vi "test-MecaDrvPoseEst2-Test2.vi"(8 "error in (no error)":errorcluster) -> (0 "error out":errorcluster, 3 "Test Passed":bool)   [LabVIEW 2019]
uses:
  <vilib>/Rock Robotics/WPI/ThirdParty/JAS_Junk/TrajLib/Rotation2d_CreateAngle.vi
  <vilib>/Rock Robotics/WPI/ThirdParty/JAS_Junk/TrajLib/MatBuilder_Create.vi
  <vilib>/Rock Robotics/WPI/ThirdParty/JAS_Junk/TrajLib/Pose2d_TransformBy.vi
  <vilib>/Rock Robotics/WPI/ThirdParty/JAS_Junk/TrajLib/Translation2d_RotateBy.vi
  <vilib>/Rock Robotics/WPI/ThirdParty/JAS_Junk/TrajLib/Translation2d_Plus.vi
  <vilib>/Rock Robotics/WPI/ThirdParty/JAS_Junk/TrajLib/Rotation2d_Plus.vi
  <vilib>/Rock Robotics/WPI/ThirdParty/JAS_Junk/TrajLib/Pose2d_New_TRRO.vi
  <vilib>/Rock Robotics/WPI/ThirdParty/JAS_Junk/TrajLib/Rotation2d_RotateBy.vi
  <vilib>/Rock Robotics/WPI/ThirdParty/JAS_Junk/TrajLib/Rotation2d_CreateXY.vi
  <vilib>/Rock Robotics/WPI/ThirdParty/JAS_Junk/TrajLib/Util_CalcDist.vi
  <vilib>/Rock Robotics/WPI/ThirdParty/JAS_Junk/TrajLib/Trajectory_Library.lvlib
panel:
  out "max x error":dbl
  out "max y err":dbl
  out "Y Error":dbl[](array[numeric])
  out "X error":dbl[](array[numeric])
  out "Total":i32
  out "Total passed":i32
  out "Sub error":bool
  out "End Y pos passed":bool
  out "End X pos passed":bool
  out "AddVisionCount":i32
  out "TotalTImeSecs 2":dbl
  out "BenchProcessing \nTimer Per Pass":dbl
  out "BenchTotalTime":dbl
  out "BenchTotalPasses":dbl
  out "MaxErrPassed":bool
  out "MeanPassed":bool
  out "ErrorSumNormalized":dbl
  out "Error Sum":dbl
  out "Max Error":dbl
  out "VIsionMeasCount":i32
  out "TotalTImeSecs":dbl
  out "Position Graph":cluster{dbl[], dbl[]}[](graph)
  out "PoseEst2NewErr":errorcluster
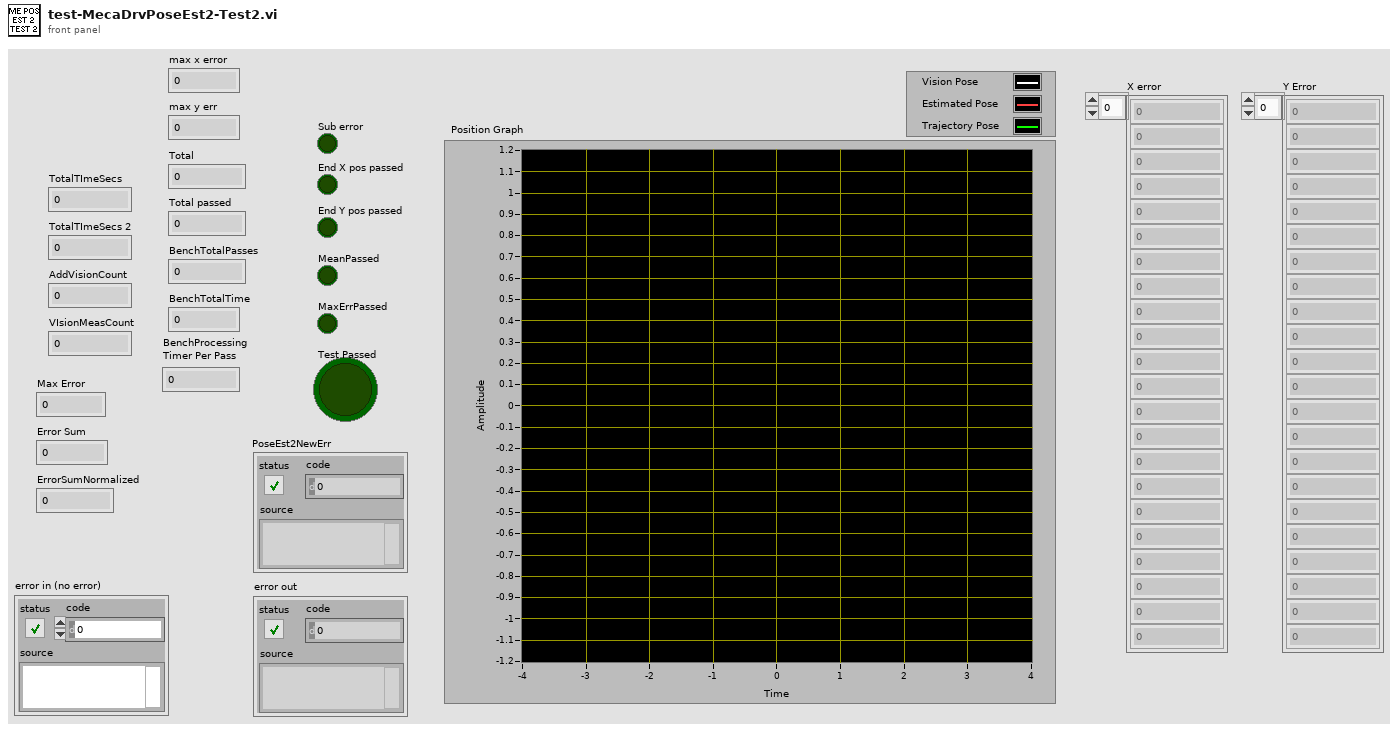
[diagram p1: front panel]
types:
  T1 = typedef "Trajectory_Library.lvlib/TRANSLATION2D.ctl" = cluster{"X":dbl, "Y":dbl}
  T2 = typedef "Trajectory_Library.lvlib/MECA_DRIVE_KINEMATICS.ctl" = cluster{"FrontLeft":T1, "FrontRight":T1, "RearLeft":T1, "RearRight":T1, "InverseKinematics":T3, "ForwardKinematics":T3, "PrevCoR":T1}
  T3 = typedef "NI_Matrix.lvlib/RealMatrix.ctl" = dbl[][]
  T4 = typedef "Trajectory_Library.lvlib/MECA_WHEEL_POSITIONS.ctl" = cluster{"FrontLeft":dbl, "FrontRight":dbl, "RearLeft":dbl, "RearRight":dbl, "P":bool}
  T5 = typedef "Trajectory_Library.lvlib/POSE2D.ctl" = cluster{"TRANSLATION":T1, "ROTATION":T6}
  T6 = typedef "Trajectory_Library.lvlib/ROTATION2D.ctl" = cluster{"VALUE":dbl, "COS":dbl, "SIN":dbl}
  T7 = typedef "Trajectory_Library.lvlib/TRAJ_CONFIG.ctl" = cluster{"MaxVelocity":dbl, "Max Acceleration":dbl, "StartVelocity":dbl, "End Velocity":dbl, "Reversed":bool, "Constraints":variant[]}
  T8 = typedef "Trajectory_Library.lvlib/MECA_DRIVE_POSE_EST2.ctl" = cluster{"M_Vision_K":T3, "m_nominal_dT":dbl, "m_PrevTime_Sec":dbl, "Pose_Buffer":T9, "Meca_Drive_Odom":T10, "M_Q":T3}
  T9 = typedef "Trajectory_Library.lvlib/TIME_INTERPOLATABLE_VARIANT.ctl" = cluster{"TimeStamps":dbl[], "DataArray":variant[], "Min_TimeStamp":dbl, "Max_TimeStamp":dbl, "ItemCount":i32, "MaxBufferTime":dbl}
  T10 = typedef "Trajectory_Library.lvlib/MECA_DRIVE_ODOMETRY.ctl" = cluster{"POSE":T5, "GyroOffset":T6, "PreviousAngle":T6, "Kinematics":T2, "PreviousWheelPositions":T4}
  T11 = typedef "Trajectory_Library.lvlib/TRAJECTORY.ctl" = cluster{"TotalTImeSecs":dbl, "States":T12[]}
  T12 = typedef "Trajectory_Library.lvlib/TRAJ_STATE.ctl" = cluster{"TimeSeconds":dbl, "Velocity":dbl, "Acceleration":dbl, "POSE":T5, "Curvature":dbl}
  T13 = typedef "Trajectory_Library.lvlib/TRANSFORM2D.ctl" = cluster{"TRANSLATION":T1, "ROTATION":T6, "xF":bool}
  T14 = cluster{"MaxErrPassed":bool, "MeanPassed":bool, "Error Sum":dbl, "ErrorSumNormalized":dbl, "Max Error":dbl, "AddVisionCount":i32, "VIsionApplyCount":i32, "BenchTotalPasses":dbl, "BenchTotalTime":dbl, "BenchProcessing \nTimer Per Pass":dbl, "TotalTImeSecs":dbl, "End X pos passed":bool, "End Y pos passed":bool, "Sub error":bool, "End X Dev":dbl, "End Y Dev":dbl}
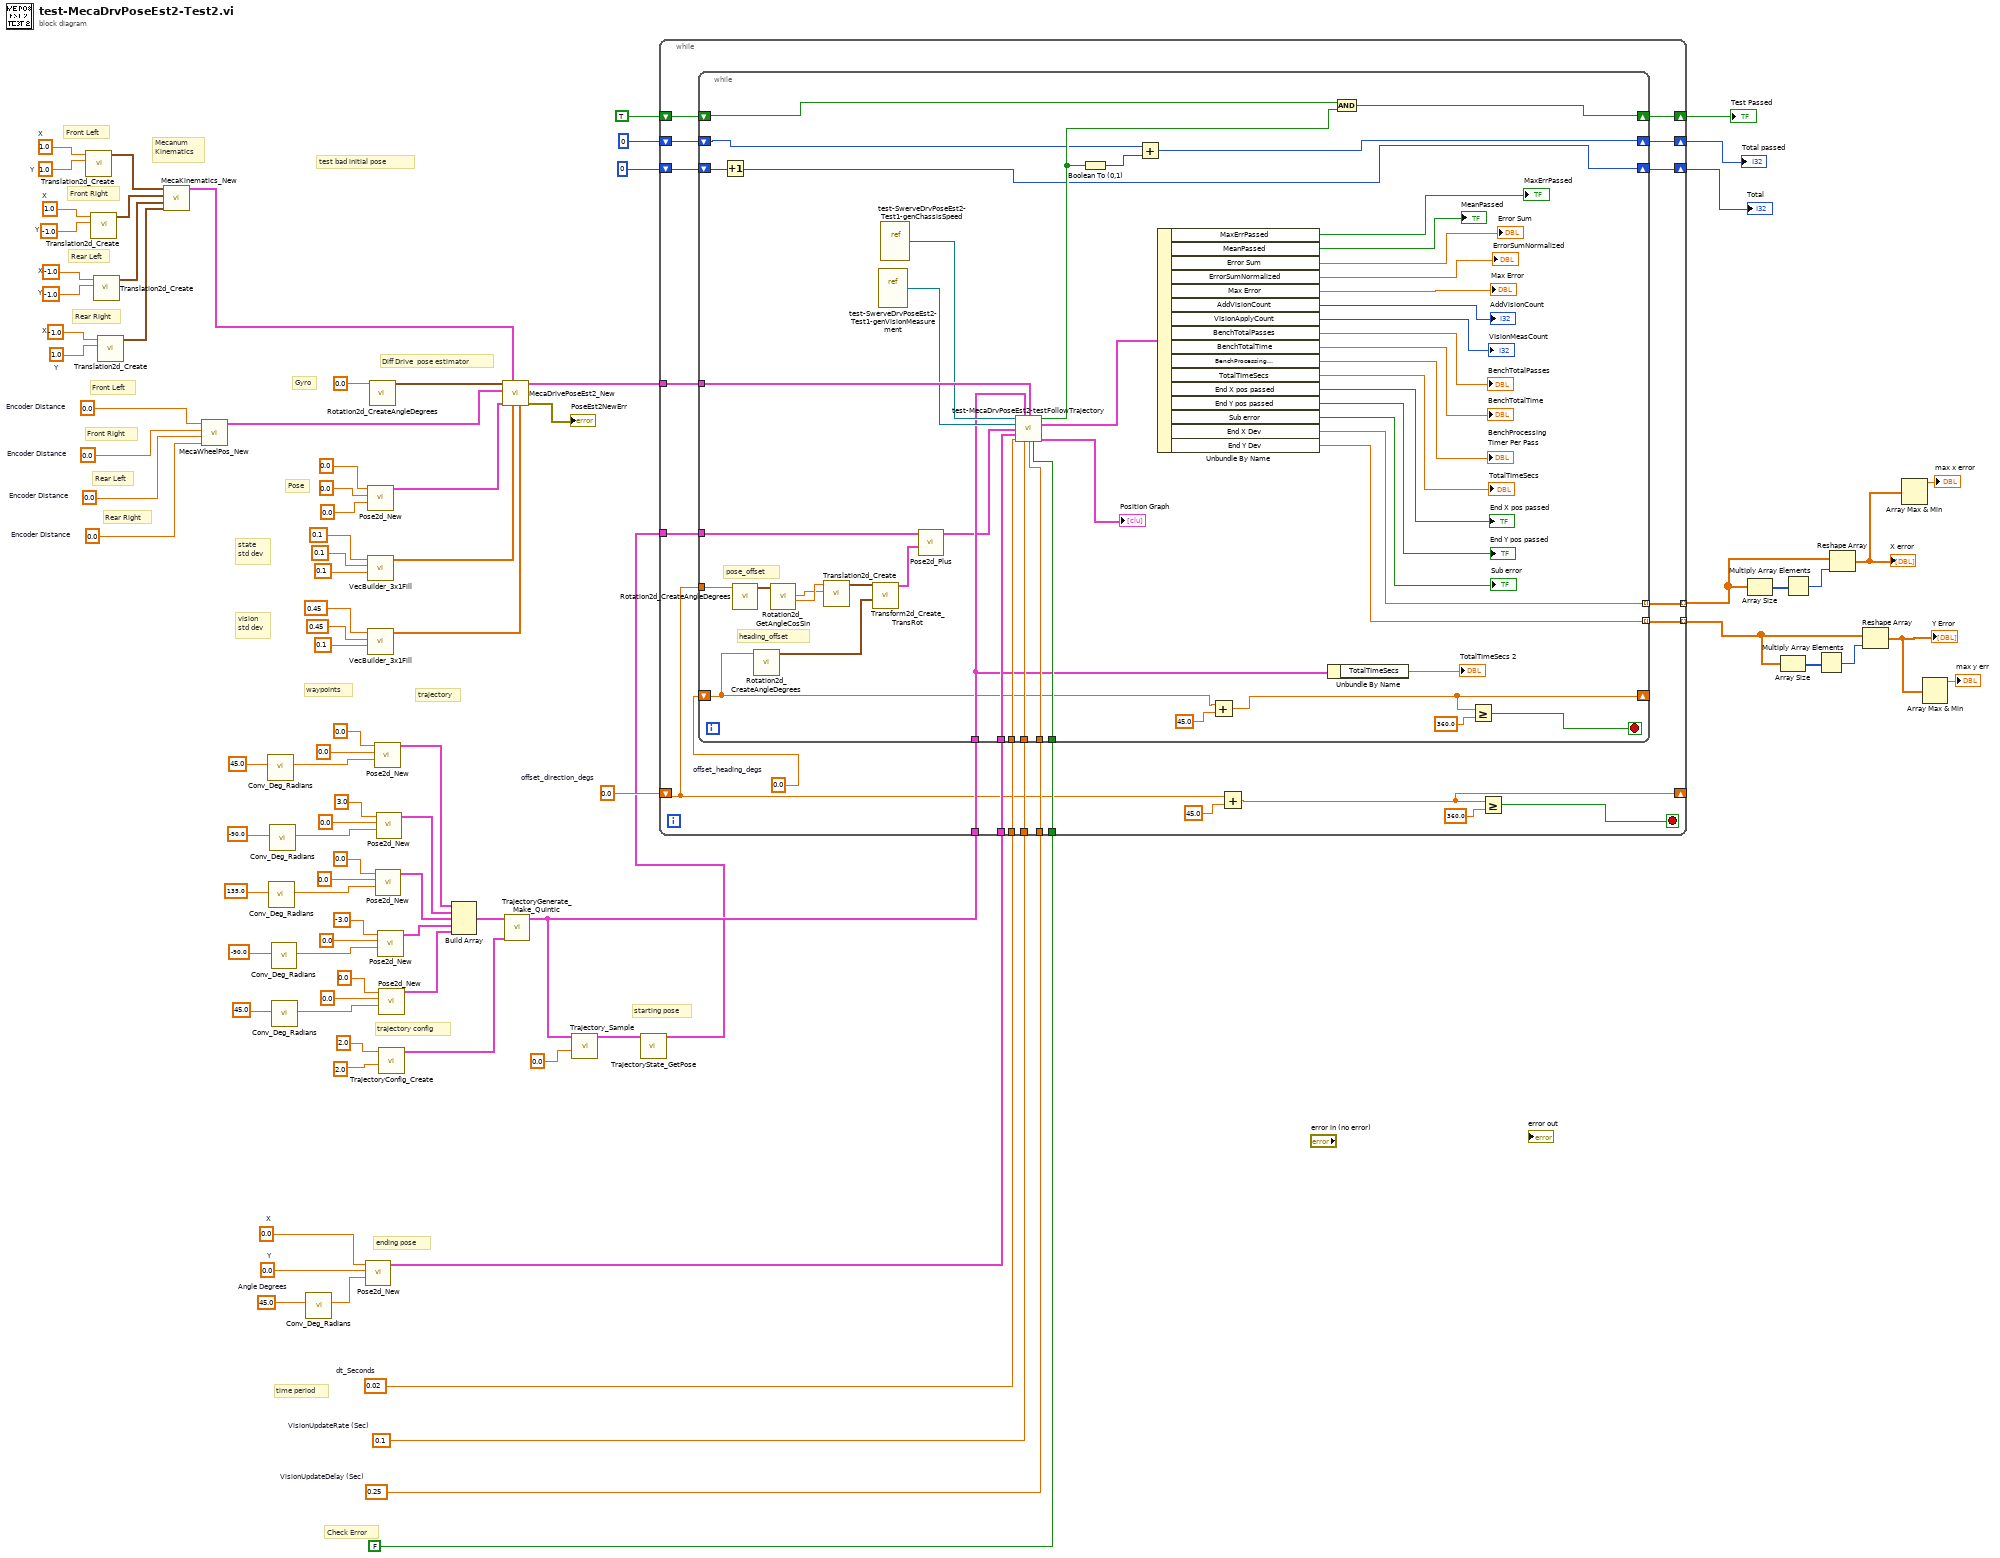
[diagram p0: block diagram]
diagram:
  w10 = -1.0  # X
  w9 = 1.0  # Y
  w8 = -1.0  # X
  w7 = -1.0  # Y
  w6 = 1.0  # X
  w5 = -1.0  # Y
  w4 = 1.0  # X
  w3 = 1.0  # Y
  w15 = 0.0  # Encoder Distance
  w16 = 0.0  # Encoder Distance
  w17 = 0.0  # Encoder Distance
  w18 = 0.0  # Encoder Distance
  w36 = 0.0  # offset_direction_degs
  w41 = 0.25  # VisionUpdateDelay (Sec)
  w42 = 0.1  # VisionUpdateRate (Sec)
  w47 = 0.0  # X
  w46 = 0.0  # Y
  w44 = 45.0  # Angle Degrees
  w48 = 0.02  # dt_Seconds
  # "Mecanum\nKinematics"
  # "Rear Right"
  # "Rear Left"
  # "Front Right"
  # "Front Left"
  # "Front Left"
  # "Rear Right"
  # "Rear Left"
  # "Front Right"
  # "test bad initial pose"
  # "starting pose"
  # "Check Error"
  # "ending pose"
  # "state \nstd dev"
  # "time period"
  # "vision \nstd dev"
  # "Pose"
  # "Gyro"
  # "Diff Drive  pose estimator"
  # "trajectory config"
  # "trajectory"
  # "waypoints"
  n1 = call <vilib>:"Translation2d_Create.vi"("Y"=w3, "X"=w4) -> ("TRANSLATION"=w11:T1)  [unwired: 9 in]
  n2 = call <vilib>:"Translation2d_Create.vi"("Y"=w5, "X"=w6) -> ("TRANSLATION"=w12:T1)  [unwired: 9 in]
  n3 = call <vilib>:"Translation2d_Create.vi"("Y"=w7, "X"=w8) -> ("TRANSLATION"=w13:T1)  [unwired: 9 in]
  n4 = call <vilib>:"Translation2d_Create.vi"("Y"=w9, "X"=w10) -> ("TRANSLATION"=w14:T1)  [unwired: 9 in]
  n5 = call <vilib>:"MecaKinematics_New.vi"("RearRight"=w14, "RearLeft"=w13, "FrontRight"=w12, "FrontLeft"=w11) -> ("MECA_DRIVE_KINEMATICS"=w1:T2)  [unwired: 7 in]
  n6 = call <vilib>:"MecaWheelPos_New.vi"("RearRightPosition"=w15, "RearLeftPosition"=w16, "FrontRightPosition"=w17, "FrontLeftPosition"=w18) -> ("MECA_WHEEL_POSITIONS"=w2:T4)  [unwired: 7 in]
  n7 = call <vilib>:"Conv_Deg_Radians.vi"("Degress"=45.0 ("Heading")) -> ("Radians"=w70:dbl)  [unwired: 10 in]
  n8 = call <vilib>:"Conv_Deg_Radians.vi"("Degress"=135.0 ("Heading")) -> ("Radians"=w78:dbl)  [unwired: 10 in]
  n9 = call <vilib>:"Conv_Deg_Radians.vi"("Degress"=-90.0 ("Heading")) -> ("Radians"=w74:dbl)  [unwired: 10 in]
  n10 = call <vilib>:"Conv_Deg_Radians.vi"("Degress"=-90.0 ("Heading")) -> ("Radians"=w82:dbl)  [unwired: 10 in]
  n11 = call <vilib>:"Conv_Deg_Radians.vi"("Degress"=45.0 ("Heading")) -> ("Radians"=w86:dbl)  [unwired: 10 in]
  n12 = call <vilib>:"Conv_Deg_Radians.vi"("Degress"=w44) -> ("Radians"=w45:dbl)  [unwired: 10 in]
  n13 = call <vilib>:"Pose2d_New.vi"("Heading"=w45, "Y"=w46, "X"=w47) -> ("out POSe"=w43:T5)  [unwired: 8 in]
  n14 = call <vilib>:"Pose2d_New.vi"("Heading"=0.0, "Y"=0.0, "X"=0.0) -> ("out POSe"=w56:T5)  [unwired: 8 in]
  n15 = call <vilib>:"VecBuilder_3x1Fill.vi"("R2"=0.1 ("element"), "R1"=0.1 ("element"), "R0"=0.1 ("element")) -> ("output matrix"=w51:T3)  [unwired: 8 in]
  n16 = call <vilib>:"VecBuilder_3x1Fill.vi"("R2"=0.1 ("element"), "R1"=0.45 ("element"), "R0"=0.45 ("element")) -> ("output matrix"=w50:T3)  [unwired: 8 in]
  n17 = call <vilib>:"Rotation2d_CreateAngleDegrees.vi"("Angle_Degrees"=0.0) -> ("ROTATION"=w55:T6)  [unwired: 10 in]
  n18 = call <vilib>:"Pose2d_New.vi"("Heading"=w70, "Y"=0.0, "X"=0.0) -> ("out POSe"=w69:T5)  [unwired: 8 in]
  n19 = call <vilib>:"Pose2d_New.vi"("Heading"=w78, "Y"=0.0, "X"=0.0) -> ("out POSe"=w66:T5)  [unwired: 8 in]
  n20 = call <vilib>:"Pose2d_New.vi"("Heading"=w74, "Y"=0.0, "X"=3.0) -> ("out POSe"=w67:T5)  [unwired: 8 in]
  n21 = call <vilib>:"Pose2d_New.vi"("Heading"=w82, "Y"=0.0, "X"=-3.0) -> ("out POSe"=w65:T5)  [unwired: 8 in]
  n22 = call <vilib>:"Pose2d_New.vi"("Heading"=w86, "Y"=0.0, "X"=0.0) -> ("out POSe"=w91:T5)  [unwired: 8 in]
  n23 = call <vilib>:"TrajectoryConfig_Create.vi"("MaxAcceleration"=2.0, "MaxVelocity"=2.0) -> ("TRAJECTORY_CONFIG"=w88:T7)  [unwired: 9 in]
  n24 = Build Array(w69, w67, w66, w65, w91) -> (w89:T5[])
  n25 = call <vilib>:"MecaDrivePoseEst2_New.vi"("VisionMeasurementStdDevs"=w50, "StateStdDevs"=w51, "MECA_DRIVE_KINEMATICS"=w1, "InitialPose"=w56, "Module Positions"=w2, "gyroAngle"=w55) -> ("Error"=→"PoseEst2NewErr":errorcluster, "MecaDrivePoseEstimate"=w49:T8)  [unwired: 4 in]
  n26 = call <vilib>:"TrajectoryGenerate_Make_Quintic.vi"("traj_config"=w88, "waypointPOSE"=w89) -> ("TRAJECTORY"=w39:T11)  [unwired: 8 in, 1 out]
  n27 = call <vilib>:"Trajectory_Sample.vi"("Time"=0.0, "InputTRAJECTORY"=w39) -> ("OutputTRAJ_STATE"=w37:T12)  [unwired: 9 in]
  n28 = call <vilib>:"TrajectoryState_GetPose.vi"("TRAJ_STATE"=w37) -> ("TrajStatePose"=w35:T5)  [unwired: 10 in]
  n29 = while {
    tunnel: w49 -> [w115]
    tunnel: w48 -> [w114]
    tunnel: w43 -> [w113]
    tunnel: w42 -> [w112]
    tunnel: w41 -> [w111]
    tunnel: FALSE -> [w110]
    tunnel: w39 -> [w109]
    shift-right: [w104] -> _
    shift-left: w36 -> [w102]
    tunnel: w35 -> [w103]
    shift-right: [w100] -> w33
    shift-left: TRUE -> [w101]
    shift-right: [w98] -> w31
    shift-left: 0 -> [w99]
    shift-right: [w96] -> w29
    shift-left: 0 -> [w97]
    tunnel: [w95] -> w27 mode=indexing
    tunnel: [w94] -> w23 mode=indexing
    stop <- w106 stop-if-true
    w105 = 0.0  # offset_heading_degs
    n30 = while {
      tunnel: w115 -> [w165]
      tunnel: w114 -> [w164]
      tunnel: w113 -> [w163]
      tunnel: w112 -> [w162]
      tunnel: w111 -> [w161]
      tunnel: w110 -> [w159]
      tunnel: w109 -> [w141]
      shift-right: [w136] -> _
      shift-left: w105 -> [w134]
      tunnel: w103 -> [w127]
      tunnel: w102 -> [w132]
      shift-right: [w124] -> w100
      shift-left: w101 -> [w125]
      shift-right: [w120] -> w98
      shift-left: w99 -> [w122]
      shift-right: [w118] -> w96
      shift-left: w97 -> [w119]
      tunnel: [w117] -> w95 mode=indexing
      tunnel: [w116] -> w94 mode=indexing
      stop <- w137 stop-if-true
      # "heading_offset"
      # "pose_offset"
      n31 = Increment(x=w119) -> (x+1=w118:i32)
      n32 = call <vilib>:"Rotation2d_CreateAngleDegrees.vi"("Angle_Degrees"=w132) -> ("ROTATION"=w133:T6)  [unwired: 10 in]
      n33 = call <vilib>:"Rotation2d_CreateAngleDegrees.vi"("Angle_Degrees"=w134) -> ("ROTATION"=w129:T6)  [unwired: 10 in]
      n34 = call <vilib>:"Rotation2d_GetAngleCosSin.vi"("in ROTATION"=w133) -> ("Cosine"=w131:dbl, "Sine"=w130:dbl)  [unwired: 8 in, 1 out]
      n35 = call <vilib>:"Translation2d_Create.vi"("Y"=w130, "X"=w131) -> ("TRANSLATION"=w135:T1)  [unwired: 9 in]
      n36 = call <vilib>:"Transform2d_Create_TransRot.vi"("ROTATION"=w129, "TRANSLATION"=w135) -> ("TRANSFORM"=w128:T13)  [unwired: 9 in]
      n37 = vi-ref "test-SwerveDrvPoseEst2-Test1-genVisionMeasurement.vi"() -> (w157:refnum<vi>)
      n38 = vi-ref "test-SwerveDrvPoseEst2-Test1-genChassisSpeed.vi"() -> (w158:refnum<vi>)
      n39 = call <vilib>:"Pose2d_Plus.vi"("other TRANSFORM"=w128, "in POSE"=w127) -> ("out POSE"=w126:T5)  [unwired: 9 in]
      n40 = call "test-MecaDrvPoseEst2-testFollowTrajectory.vi"("chassisSpeedsGenerator"=w158, "TRAJECTORY"=w141, "MecaDrivePoseEstimate2"=w165, "genVisionMeasurement"=w157, "StartingPose"=w126, "EndingPose"=w163, "dt_Seconds"=w164, "VisionUpdateRate"=w162, "VisionUpdateDelay"=w161, "CheckError"=w159) -> ("Test Passed"=w123:bool, "Output Data"=w155:T14, "DataForGraph"=→"Position Graph":cluster{dbl[], dbl[]}[])  [unwired: 3 in]
      n41 = Boolean To (0,1)(Boolean=w123) -> (0, 1=w121:i16)
      n42 = Add(x=w122, y=w121) -> (x+y=w120:i32)
      n43 = Unbundle By Name(w155) -> ("MaxErrPassed"=→"MaxErrPassed":bool, "MeanPassed"=→"MeanPassed":bool, "Error Sum"=→"Error Sum":dbl, "ErrorSumNormalized"=→"ErrorSumNormalized":dbl, "Max Error"=→"Max Error":dbl, "AddVisionCount"=→"AddVisionCount":i32, "VIsionApplyCount"=→"VIsionMeasCount":i32, "BenchTotalPasses"=→"BenchTotalPasses":dbl, "BenchTotalTime"=→"BenchTotalTime":dbl, "BenchProcessing \nTimer Per Pass"=→"BenchProcessing \nTimer Per Pass":dbl, "TotalTImeSecs"=→"TotalTImeSecs":dbl, "End X pos passed"=→"End X pos passed":bool, "End Y pos passed"=→"End Y pos passed":bool, "Sub error"=→"Sub error":bool, "End X Dev"=w117:dbl, "End Y Dev"=w116:dbl)
      n44 = Add(x=w134, y=45.0) -> (x+y=w136:dbl)
      n45 = Unbundle By Name(w141) -> ("TotalTImeSecs"=→"TotalTImeSecs 2":dbl)
      n46 = And(x=w125, y=w123) -> (x .and. y?=w124:bool)
      n47 = Greater Or Equal?(x=w136, y=360.0) -> (x >= y?=w137:bool)
    }
    n48 = Add(x=w102, y=45.0) -> (x+y=w104:dbl)
    n49 = Greater Or Equal?(x=w104, y=360.0) -> (x >= y?=w106:bool)
  }
  "Test Passed" <- w33
  "Total passed" <- w31
  "Total" <- w29
  n50 = Array Size(array=w27) -> (size(s)=w28:i32[])
  n51 = Array Size(array=w23) -> (size(s)=w25:i32[])
  n52 = Multiply Array Elements(1:w28) -> (0:w26:i32)
  n53 = Multiply Array Elements(1:w25) -> (0:w24:i32)
  n54 = Reshape Array(w27, w26) -> (w22:dbl[])
  "X error" <- w22
  n55 = Reshape Array(w23, w24) -> (w21:dbl[])
  "Y Error" <- w21
  n56 = Array Max & Min(array=w22) -> (max value=→"max x error":dbl)  [unwired: 3 out]
  n57 = Array Max & Min(array=w21) -> (max value=→"max y err":dbl)  [unwired: 3 out]
